vi "VSI Init SPI.vi"(9 "pInitConfig":T1, 10 "DevIndex":i32, 11 "DevType":i32) -> (1 "pInitConfig out":T1, 3 "function return":i32)   [LabVIEW 2010, in "ControlSPI.lvlib"]
doc: "int WINAPI VSI_InitSPI(int DevType, int DevIndex, PVSI_INIT_CONFIG pInitConfig);"
uses:
  ControlSPI.lvlib
  ControlSPI/Ginkgo_Driver.dll
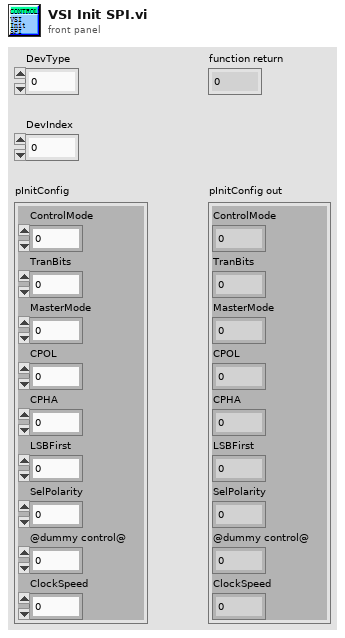
[diagram p1: front panel]
types:
  T1 = cluster{"ControlMode":u8, "TranBits":u8, "MasterMode":u8, "CPOL":u8, "CPHA":u8, "LSBFirst":u8, "SelPolarity":u8, "@dummy control@":i8, "ClockSpeed":u32}
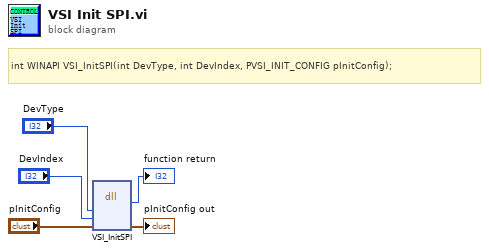
[diagram p0: block diagram]
diagram:
  # "int WINAPI VSI_InitSPI(int DevType, int DevIndex, PVSI_INIT_CONFIG pInitConfig);"
  n1 = dll-call lib="E:/Project/vt_ginkgo/truck/Ginkgo Driver/vs2010/Ginkgo_USB-I2C&SPI&CAN_API_v2.0.3.3/lib/labview_32bit/ControlSPI/Ginkgo_Driver.*" fn="VSI_InitSPI"("DevType"="DevType", "DevIndex"="DevIndex", "pInitConfig"="pInitConfig") -> (→"function return":i32, "pInitConfig"=→"pInitConfig out":T1)  [unwired: 5 in, 2 out]
